vi "CalGas aufschalten Paccar.vi"() -> (3 "Cluster":T1)   [LabVIEW 2020, in "Allgemein.lvlib"]
uses:
  Allgemein.lvlib
  FGV Analysator aktiv.ctl
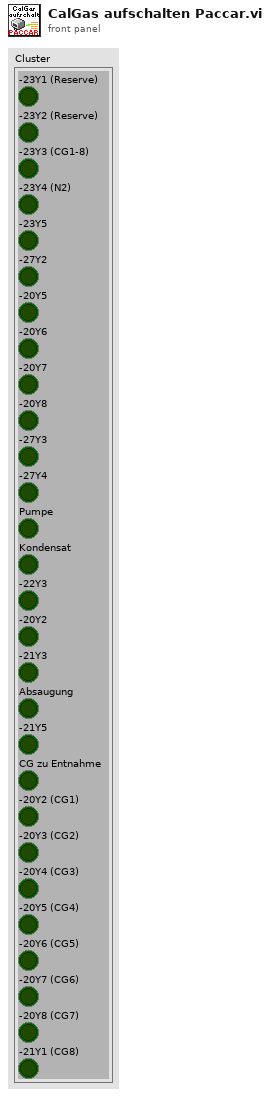
[diagram p1: front panel]
types:
  T1 = cluster{"-23Y1 (Reserve)":bool, "-23Y2 (Reserve)":bool, "-23Y3 (CG1-8)":bool, "-23Y4 (N2)":bool, "-23Y5":bool, "-27Y2":bool, "-20Y5":bool, "-20Y6":bool, "-20Y7":bool, "-20Y8":bool, "-27Y3":bool, "-27Y4":bool, "Pumpe":bool, "Kondensat":bool, "-22Y3":bool, "-20Y2":bool, "-21Y3":bool, "Absaugung":bool, "-21Y5":bool, "CG zu Entnahme":bool, "-20Y2 (CG1)":bool, "-20Y3 (CG2)":bool, "-20Y4 (CG3)":bool, "-20Y5 (CG4)":bool, "-20Y6 (CG5)":bool, "-20Y7 (CG6)":bool, "-20Y8 (CG7)":bool, "-21Y1 (CG8)":bool}
  T2 = typedef "Allgemein.lvlib/FGV Analysator aktiv.ctl" = enum16{"lesen", "Analysator", "CG Aufschaltung", "KAL Zustand", "AutaKal GT?"}
  T3 = typedef "CalGas Aufschaltung.lvlib/Aufschaltung CalGas.ctl" = cluster{"Kalibriergas":T4, "Aufschaltpunkt":T5, "Analysator":T6}
  T4 = typedef "Auswahlfeld.ctl" = u16
  T5 = typedef "CalGas Aufschaltung.lvlib/Auswahl Aufschaltpunkt.ctl" = enum16{"über Filterblock", "Analysator direkt", "über PNS", "Entnahme", "Gasdivider"}
  T6 = typedef "CalGas Aufschaltung.lvlib/Auswahl Analysator.ctl" = enum16{"FT-IR", "FID", "PMA", "PMA/FID/FT-IR"}
  T7 = typedef "Status Analysatoren.lvlib/Status Analysatoren_Anzeige.ctl" = cluster{"FT-IR":bool, "FID":bool, "PMA":bool}
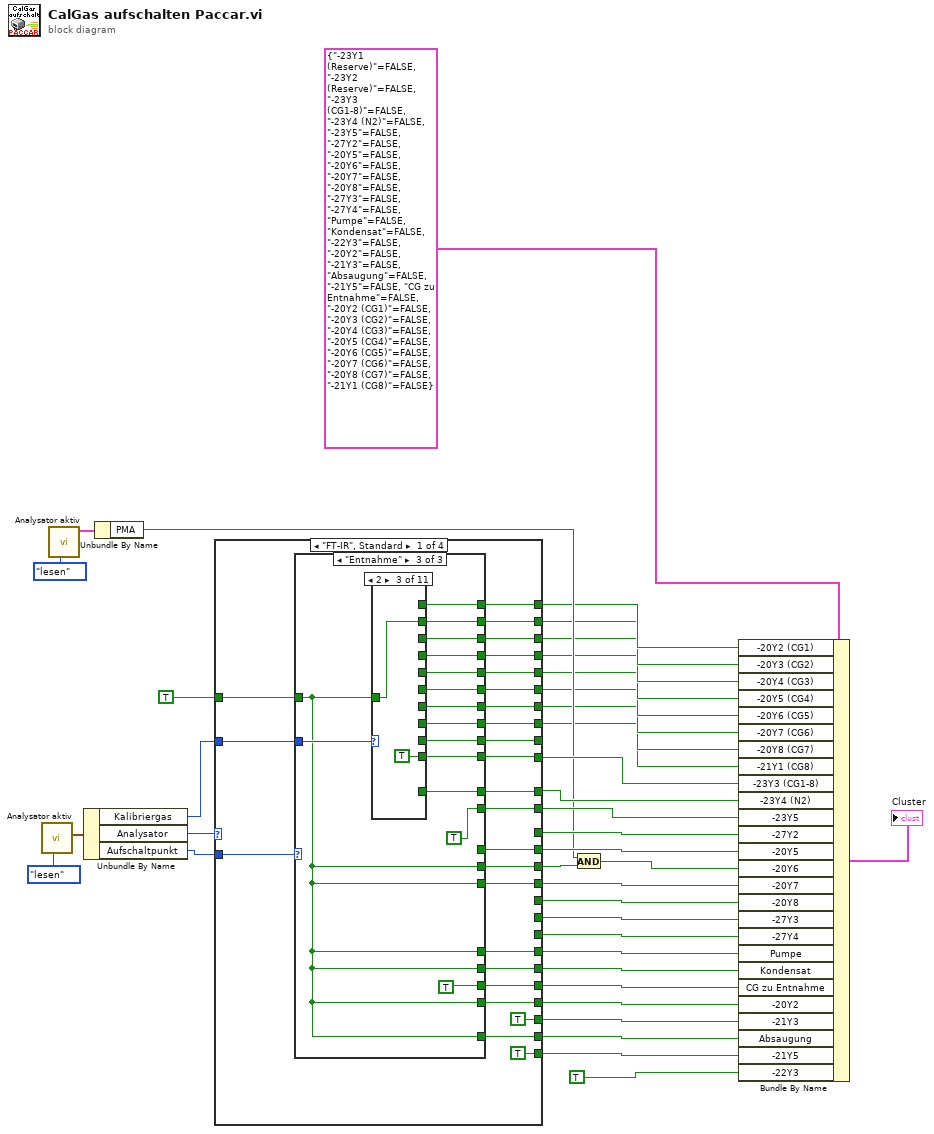
[diagram p0: block diagram]
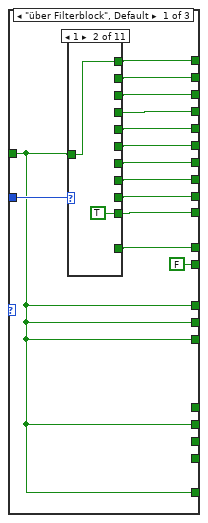
[diagram p2: hidden frame]
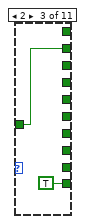
[diagram p4: hidden frame]
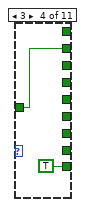
[diagram p5: hidden frame]
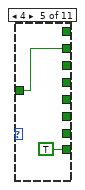
[diagram p6: hidden frame]
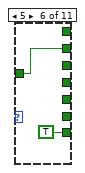
[diagram p7: hidden frame]
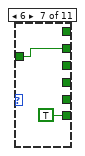
[diagram p8: hidden frame]
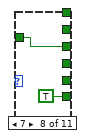
[diagram p9: hidden frame]
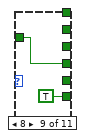
[diagram p10: hidden frame]
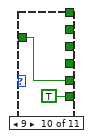
[diagram p11: hidden frame]
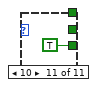
[diagram p12: hidden frame]
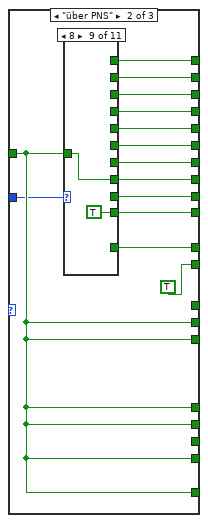
[diagram p13: hidden frame]
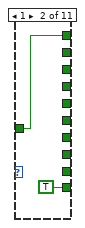
[diagram p15: hidden frame]
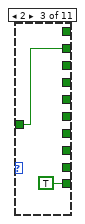
[diagram p16: hidden frame]
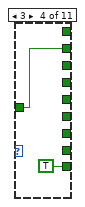
[diagram p17: hidden frame]
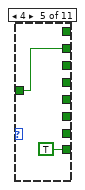
[diagram p18: hidden frame]
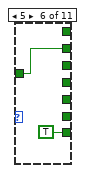
[diagram p19: hidden frame]
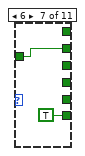
[diagram p20: hidden frame]
diagram:
  n1 = call "Analysator aktiv.vi"("Aktion"=FGV_Analysator_aktiv."lesen") -> ("Aufschaltung CalGas"=w37:T3)  [unwired: 7 in, 3 out]
  n2 = call "Analysator aktiv.vi"("Aktion"=FGV_Analysator_aktiv."lesen") -> ("Status Analysatoren"=w15:T7)  [unwired: 7 in, 3 out]
  n3 = Unbundle By Name(w37) -> ("Kalibriergas"=w21:T4, "Analysator"=w36:T6, "Aufschaltpunkt"=w35:T5)
  n4 = Unbundle By Name(w15) -> ("PMA"=w13:bool)
  n5 = case shown="\"FT-IR\", Standard" w36 {
    tunnel: w35 -> [w63 w185 w245 w291]
    tunnel: TRUE -> [w62 w184 w233 w279]
    tunnel: [w60 w182 w243 w289] -> _
    tunnel: [w39 w181 w242 w288] -> w33
    tunnel: [w59 w180 w241 w287] -> w32
    tunnel: [w58 w179 w240 w286] -> w31
    tunnel: [_ w169 _ _] -> w30
    tunnel: [w57 w178 w239 w285] -> w29
    tunnel: [w50 w173 w229 w275] -> w28
    tunnel: [w56 w177 w238 w284] -> w27
    tunnel: [_ _ w235 w281] -> w26
    tunnel: [_ w170 _ _] -> w25
    tunnel: [_ w171 _ w272] -> w24
    tunnel: [w55 w176 w237 w283] -> w23
    tunnel: [w51 w172 w228 w274] -> w22
    tunnel: w21 -> [w61 w183 w244 w290]
    tunnel: [w54 w175 w236 w282] -> w20
    tunnel: [TRUE TRUE w231 w277] -> w19
    tunnel: [w52 w168 w230 w276] -> w18
    tunnel: [TRUE w167 TRUE TRUE] -> w17
    tunnel: [w48 _ _ _] -> w11
    tunnel: [w47 _ _ _] -> w9
    tunnel: [w46 _ _ _] -> w8
    tunnel: [w45 _ _ _] -> w7
    tunnel: [w44 _ _ _] -> w6
    tunnel: [w43 _ _ _] -> w5
    tunnel: [w42 _ _ _] -> w4
    tunnel: [w41 _ _ _] -> w3
    tunnel: [w40 _ _ _] -> w2
    frame "FT-IR", Default {
      n6 = case shown="\"Entnahme\"" w63 {
        tunnel: w62 -> [w75 w110 w142]
        tunnel: w61 -> [w76 w109 w146]
        tunnel: [w66 w100 w145] -> w60
        tunnel: [w64 w98 w144] -> w59
        tunnel: [FALSE TRUE TRUE] -> w58
        tunnel: [w75 _ _] -> w57
        tunnel: [w75 w110 w142] -> w56
        tunnel: [_ w110 w142] -> w55
        tunnel: [_ w110 w142] -> w54
        tunnel: [w75 w110 w142] -> w52
        tunnel: [w75 w110 w142] -> w51
        tunnel: [w75 w110 w142] -> w50
        tunnel: [_ _ TRUE] -> w48
        tunnel: [w74 w108 w140] -> w47
        tunnel: [w73 w107 w139] -> w46
        tunnel: [w72 w106 w138] -> w45
        tunnel: [w71 w105 w137] -> w44
        tunnel: [w70 w104 w136] -> w43
        tunnel: [w69 w103 w135] -> w42
        tunnel: [w68 w102 w134] -> w41
        tunnel: [w67 w101 w133] -> w40
        tunnel: [w65 w99 w132] -> w39
        frame "über Filterblock", Default {
          n7 = case shown="1" w76 {
            tunnel: w75 -> [w78 w80 w82 w84 w86 w88 w90 w92 w94 w96 _]
            tunnel: [_ _ _ _ _ _ _ _ _ w96 _] -> w66
            tunnel: [w78 _ _ _ _ _ _ _ _ _ _] -> w64
            tunnel: [_ w80 _ _ _ _ _ _ _ _ _] -> w74
            tunnel: [_ _ w82 _ _ _ _ _ _ _ _] -> w73
            tunnel: [_ _ _ w84 _ _ _ _ _ _ _] -> w72
            tunnel: [_ _ _ _ w86 _ _ _ _ _ _] -> w71
            tunnel: [_ _ _ _ _ w88 _ _ _ _ _] -> w70
            tunnel: [_ _ _ _ _ _ w90 _ _ _ _] -> w69
            tunnel: [_ _ _ _ _ _ _ w92 _ _ _] -> w68
            tunnel: [_ _ _ _ _ _ _ _ w94 _ _] -> w67
            tunnel: [_ TRUE TRUE TRUE TRUE TRUE TRUE TRUE TRUE TRUE TRUE] -> w65
            frame 0, Default {
            }
            frame 1 {
            }
            frame 2 {
            }
            frame 3 {
            }
            frame 4 {
            }
            frame 5 {
            }
            frame 6 {
            }
            frame 7 {
            }
            frame 8 {
            }
            frame 9 {
            }
            frame 10 {
            }
          }
        }
        frame "über PNS" {
          n8 = case shown="8" w109 {
            tunnel: w110 -> [w112 w114 w116 w118 w120 w122 w124 w126 w128 w130 _]
            tunnel: [_ _ _ _ _ _ _ _ _ w130 _] -> w100
            tunnel: [w112 _ _ _ _ _ _ _ _ _ _] -> w98
            tunnel: [_ w114 _ _ _ _ _ _ _ _ _] -> w108
            tunnel: [_ _ w116 _ _ _ _ _ _ _ _] -> w107
            tunnel: [_ _ _ w118 _ _ _ _ _ _ _] -> w106
            tunnel: [_ _ _ _ w120 _ _ _ _ _ _] -> w105
            tunnel: [_ _ _ _ _ w122 _ _ _ _ _] -> w104
            tunnel: [_ _ _ _ _ _ w124 _ _ _ _] -> w103
            tunnel: [_ _ _ _ _ _ _ w126 _ _ _] -> w102
            tunnel: [_ _ _ _ _ _ _ _ w128 _ _] -> w101
            tunnel: [_ TRUE TRUE TRUE TRUE TRUE TRUE TRUE TRUE TRUE TRUE] -> w99
            frame 0, Default {
            }
            frame 1 {
            }
            frame 2 {
            }
            frame 3 {
            }
            frame 4 {
            }
            frame 5 {
            }
            frame 6 {
            }
            frame 7 {
            }
            frame 8 {
            }
            frame 9 {
            }
            frame 10 {
            }
          }
        }
        frame "Entnahme" {
          n9 = case shown="2" w146 {
            tunnel: w142 -> [w147 w149 w151 w153 w155 w157 w159 w161 w163 w165 _]
            tunnel: [_ _ _ _ _ _ _ _ _ w165 _] -> w145
            tunnel: [w147 _ _ _ _ _ _ _ _ _ _] -> w144
            tunnel: [_ w149 _ _ _ _ _ _ _ _ _] -> w140
            tunnel: [_ _ w151 _ _ _ _ _ _ _ _] -> w139
            tunnel: [_ _ _ w153 _ _ _ _ _ _ _] -> w138
            tunnel: [_ _ _ _ w155 _ _ _ _ _ _] -> w137
            tunnel: [_ _ _ _ _ w157 _ _ _ _ _] -> w136
            tunnel: [_ _ _ _ _ _ w159 _ _ _ _] -> w135
            tunnel: [_ _ _ _ _ _ _ w161 _ _ _] -> w134
            tunnel: [_ _ _ _ _ _ _ _ w163 _ _] -> w133
            tunnel: [_ TRUE TRUE TRUE TRUE TRUE TRUE TRUE TRUE TRUE TRUE] -> w132
            frame 0, Default {
            }
            frame 1 {
            }
            frame 2 {
            }
            frame 3 {
            }
            frame 4 {
            }
            frame 5 {
            }
            frame 6 {
            }
            frame 7 {
            }
            frame 8 {
            }
            frame 9 {
            }
            frame 10 {
            }
          }
        }
      }
    }
    frame "PMA" {
      n10 = case shown="\"über PNS\"" w185 {
        tunnel: w184 -> [w187 w199 w216]
        tunnel: w183 -> [w193 w209 w222]
        tunnel: [w192 w208 w221] -> w182
        tunnel: [w191 w207 w220] -> w181
        tunnel: [w190 w206 w219] -> _
        tunnel: [w189 w205 w218] -> w180
        tunnel: [FALSE FALSE TRUE] -> w179
        tunnel: [w187 _ _] -> w178
        tunnel: [w187 TRUE w216] -> w177
        tunnel: [_ _ w216] -> w176
        tunnel: [_ _ w216] -> w175
        tunnel: [w187 TRUE w216] -> w173
        tunnel: [w187 _ w216] -> w172
        tunnel: [w187 w199 w216] -> w171
        tunnel: [_ w202 _] -> w170
        tunnel: [_ w203 _] -> w169
        tunnel: [w187 w199 w216] -> w168
        tunnel: [FALSE FALSE TRUE] -> w167
        frame "über Filterblock", Default {
          n11 = case shown="1" w193 {
            tunnel: w187 -> [w194 w195 w196 w197]
            tunnel: [_ w195 _ _] -> w192
            tunnel: [_ _ w196 _] -> w191
            tunnel: [_ _ _ w197] -> w190
            tunnel: [w194 _ _ _] -> w189
            frame 0, Default {
            }
            frame 1 {
            }
            frame 2 {
            }
            frame 3 {
            }
          }
        }
        frame "Analysator direkt" {
          n12 = case shown="2" w209 {
            tunnel: w199 -> [w210 w211 w212 w213 w214]
            tunnel: [_ w211 _ _ _] -> w208
            tunnel: [_ _ _ _ w214] -> w207
            tunnel: [_ _ _ w213 _] -> w206
            tunnel: [w210 _ _ _ _] -> w205
            tunnel: [_ _ w212 _ _] -> w203
            tunnel: [_ _ w212 _ _] -> w202
            frame 0, Default {
            }
            frame 1 {
            }
            frame 2 {
            }
            frame 3 {
            }
            frame 4 {
            }
          }
        }
        frame "über PNS" {
          n13 = case shown="2" w222 {
            tunnel: w216 -> [w223 w224 w225 w226]
            tunnel: [_ w224 _ _] -> w221
            tunnel: [_ _ w225 _] -> w220
            tunnel: [_ _ _ w226] -> w219
            tunnel: [w223 _ _ _] -> w218
            frame 0, Default {
            }
            frame 1 {
            }
            frame 2 {
            }
            frame 3 {
            }
          }
        }
      }
    }
    frame "FID" {
      n14 = call "Verzoegerung.vi"("sec"=u16 12, "Startsignal"=w233) -> ("Zeit abgelaufen?"=w232:bool)  [unwired: 8 in, 1 out]
      n15 = case shown="\"über Filterblock\", Standard" w245 {
        tunnel: w233 -> [w246 w259]
        tunnel: w244 -> [w254 w267]
        tunnel: [w253 w266] -> w243
        tunnel: [w252 w265] -> w242
        tunnel: [w251 w264] -> _
        tunnel: [w250 w263] -> w241
        tunnel: [FALSE TRUE] -> w240
        tunnel: [w246 _] -> w239
        tunnel: [w246 w259] -> w238
        tunnel: [_ w259] -> w237
        tunnel: [_ w259] -> w236
        tunnel: [w248 w261] -> w235
        tunnel: w232 -> [w248 w261]
        tunnel: [w247 w260] -> w231
        tunnel: [w246 w259] -> w230
        tunnel: [w246 w259] -> w229
        tunnel: [w246 w259] -> w228
        frame "über Filterblock", Default {
          n16 = case shown="2" w254 {
            tunnel: w246 -> [w255 w256 w257 w258]
            tunnel: [_ w256 _ _] -> w253
            tunnel: [_ _ w257 _] -> w252
            tunnel: [_ _ _ w258] -> w251
            tunnel: [w255 _ _ _] -> w250
            frame 0, Default {
            }
            frame 1 {
            }
            frame 2 {
            }
            frame 3 {
            }
          }
          n17 = Not(x=w248) -> (.not. x?=w247:bool)
        }
        frame "über PNS" {
          n18 = case shown="2" w267 {
            tunnel: w259 -> [w268 w269 w270 w271]
            tunnel: [_ w269 _ _] -> w266
            tunnel: [_ _ w270 _] -> w265
            tunnel: [_ _ _ w271] -> w264
            tunnel: [w268 _ _ _] -> w263
            frame 0, Default {
            }
            frame 1 {
            }
            frame 2 {
            }
            frame 3 {
            }
          }
          n19 = Not(x=w261) -> (.not. x?=w260:bool)
        }
      }
    }
    frame "PMA/FID/FT-IR" {
      n20 = call "Verzoegerung.vi"("sec"=u16 12, "Startsignal"=w279) -> ("Zeit abgelaufen?"=w278:bool)  [unwired: 8 in, 1 out]
      n21 = case shown="\"über PNS\"" w291 {
        tunnel: w279 -> [w292 w306]
        tunnel: w290 -> [w300 w313]
        tunnel: [w299 w312] -> w289
        tunnel: [w298 w311] -> w288
        tunnel: [w297 w310] -> _
        tunnel: [w296 w309] -> w287
        tunnel: [FALSE TRUE] -> w286
        tunnel: [w292 _] -> w285
        tunnel: [w292 w306] -> w284
        tunnel: [_ w306] -> w283
        tunnel: [_ w306] -> w282
        tunnel: [w294 w305] -> w281
        tunnel: w278 -> [w294 w305]
        tunnel: [w293 w307] -> w277
        tunnel: [w292 w306] -> w276
        tunnel: [w292 w306] -> w275
        tunnel: [w292 w306] -> w274
        tunnel: [w292 w305] -> w272
        frame "über Filterblock", Default {
          n22 = case shown="0, Standard" w300 {
            tunnel: w292 -> [w301 w302 w303 w304]
            tunnel: [_ w302 _ _] -> w299
            tunnel: [_ _ w303 _] -> w298
            tunnel: [_ _ _ w304] -> w297
            tunnel: [w301 _ _ _] -> w296
            frame 0, Default {
            }
            frame 1 {
            }
            frame 2 {
            }
            frame 3 {
            }
          }
          n23 = Not(x=w294) -> (.not. x?=w293:bool)
        }
        frame "über PNS" {
          n24 = case shown="1" w313 {
            tunnel: w306 -> [w314 w315 w316 w317]
            tunnel: [_ w315 _ _] -> w312
            tunnel: [_ _ w316 _] -> w311
            tunnel: [_ _ _ w317] -> w310
            tunnel: [w314 _ _ _] -> w309
            frame 0, Default {
            }
            frame 1 {
            }
            frame 2 {
            }
            frame 3 {
            }
          }
          n25 = Not(x=w305) -> (.not. x?=w307:bool)
        }
      }
    }
  }
  n26 = And(x=w13, y=w28) -> (x .and. y?=w14:bool)
  n27 = Bundle By Name(cluster=T1 {"-23Y1 (Reserve)"=FALSE, "-23Y2 (Reserve)"=FALSE, "-23Y3 (CG1-8)"=FALSE, "-23Y4 (N2)"=FALSE, "-23Y5"=FALSE, "-27Y2"=FALSE, "-20Y5"=FALSE, "-20Y6"=FALSE, "-20Y7"=FALSE, "-20Y8"=FALSE, "-27Y3"=FALSE, "-27Y4"=FALSE, "Pumpe"=FALSE, "Kondensat"=FALSE, "-22Y3"=FALSE, "-20Y2"=FALSE, "-21Y3"=FALSE, "Absaugung"=FALSE, "-21Y5"=FALSE, "CG zu Entnahme"=FALSE, "-20Y2 (CG1)"=FALSE, "-20Y3 (CG2)"=FALSE, "-20Y4 (CG3)"=FALSE, "-20Y5 (CG4)"=FALSE, "-20Y6 (CG5)"=FALSE, "-20Y7 (CG6)"=FALSE, "-20Y8 (CG7)"=FALSE, "-21Y1 (CG8)"=FALSE} ("Cluster"), "-20Y2 (CG1)"=w9, "-20Y3 (CG2)"=w8, "-20Y4 (CG3)"=w7, "-20Y5 (CG4)"=w6, "-20Y6 (CG5)"=w5, "-20Y7 (CG6)"=w4, "-20Y8 (CG7)"=w3, "-21Y1 (CG8)"=w2, "-23Y3 (CG1-8)"=w33, "-23Y4 (N2)"=w32, "-23Y5"=w31, "-27Y2"=w30, "-20Y5"=w29, "-20Y6"=w14, "-20Y7"=w27, "-20Y8"=w26, "-27Y3"=w25, "-27Y4"=w24, "Pumpe"=w23, "Kondensat"=w22, "CG zu Entnahme"=w11, "-20Y2"=w20, "-21Y3"=w19, "Absaugung"=w18, "-21Y5"=w17, "-22Y3"=TRUE) -> (→"Cluster":T1)
